vi "Same Error.vi"() -> ()   [LabVIEW 2017, in "Assertions.Tests.lvlib" / "Assert Error Code.lvlib"]
uses:
  Assert Error Code.lvlib
  <vilib>/Utility/error.llb/Error Cluster From Error Code.vi
  src/Transparent Assertions/Constraints/IsEqual/Create.vi
  <vilib>/ErrorRing/Error Ring.xnode
  src/Transparent Assertions/Constraints/IsEqual/IsEqual.lvclass
  src/Transparent Assertions/Assertions/Assertions.lvlib
panel:
  out "error out":errorcluster
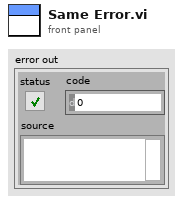
[diagram p1: front panel]
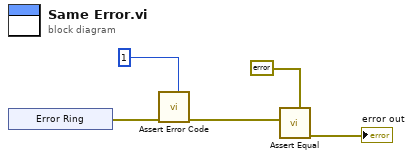
[diagram p0: block diagram]
diagram:
  n1 = xnode "Error Ring"() -> ("error out"=w4:errorcluster)
  n2 = call "Assert Error Code.vi"("Expected"=1, "error in (no error)"=w4) -> ("error out"=w2:errorcluster)  [unwired: 9 in]
  n3 = call "Assert Equal.vi"("Expected"=errorcluster {"status"=FALSE, "code"=0, "source"=""} ("error constant"), "Actual"=w2) -> ("error out"=→"error out":errorcluster)  [unwired: 9 in]
